vi "getFileExtPreference.vi"() -> (3 "Suffix to add":string)   [LabVIEW 2022 SP3]
uses:
  Setup_Filetype.ctl
panel:
  out "readingFrom":path
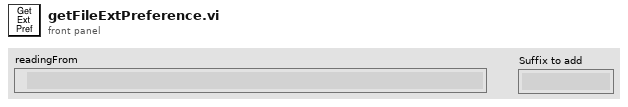
[diagram p1: front panel]
types:
  T1 = typedef "Setup_Filetype.ctl" = enum16{"Measurement Setups", "Calibration Setups", "General", "Results File Plotter Setups", "Speed Calib Tweaks"}
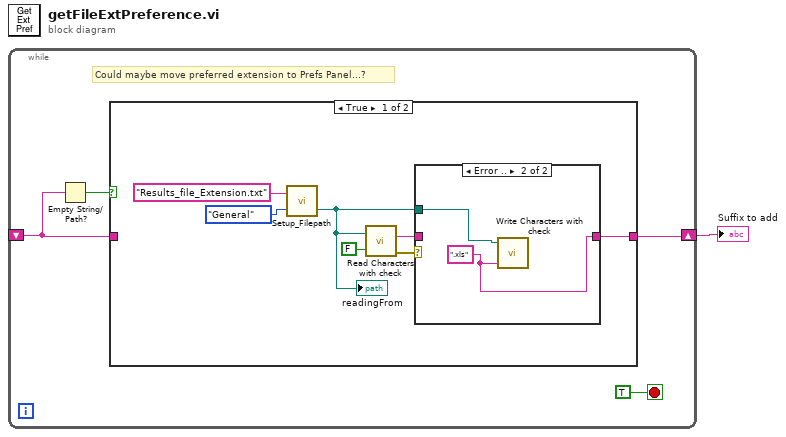
[diagram p0: block diagram]
diagram:
  n1 = while {
    shift-right: [w3] -> w1
    shift-left: _ -> [w2]
    stop <- TRUE stop-if-true
    # "Could maybe move preferred extension to Prefs Panel...?"
    n2 = Empty String/Path?(string/path=w2) -> (empty?=w4:bool)
    n3 = case shown="True" w4 {
      tunnel: [w10 w16] -> w3
      tunnel: w2 -> [_ w16]
      frame True {
        n4 = call "Setup_Filepath.vi"("Setup File Type"=Setup_Filetype."General", "Filename in"="Results_file_Extension.txt" ("name or relative path")) -> ("Filename Out"=w9:path)  [unwired: 1 out]
        "readingFrom" <- w9
        n5 = call "Read Characters with check.vi"("Call EnFlo Error Handler?"=FALSE, "file (use dialog)"=w9) -> ("error out"=w7:errorcluster, "Read String"=w8:string)
        n6 = case shown="Error .." w7 {
          tunnel: [w13 w14] -> w10
          tunnel: w8 -> [w13 _]
          tunnel: w9 -> [_ w15]
          frame No Error {
          }
          frame Error {
            w14 = ".xls" ("Suffix to add")
            n7 = call "Write Characters with check.vi"("String to Write"=w14, "file (use dialog)"=w15) -> ()  [unwired: 2 in, 1 out]
          }
        }
      }
      frame False {
      }
    }
  }
  "Suffix to add" <- w1
